vi "Configuration Keys.vi"(8 "error in":errorcluster, 11 "PowerSupply in":refnum<class "PowerSupply.lvclass">) -> (0 "error out":errorcluster, 2 "Required Keys":string[](array[string]), 3 "PowerSupply out":refnum<class "PowerSupply.lvclass">)   [LabVIEW 2019, in "PowerSupply.lvlib" / "PowerSupply.lvclass"]
doc: "Configuration Keys is a dynamic dispatch VI that reads a full inheritance chain's required key list.\n\nThis means each instrument must override this vi, and call the parent method . The end result is a comprehensive list of required keys that must be present in an instrument's config.ini file to correctly function."
uses:
  Library/PowerSupply.lvclass
  Custom Controls/Configuration Keys.ctl
  builds/Instruments/Instruments.lvlibp/Library/Instruments.lvclass
panel:
  in  "Configuration Keys":T1=enum."Number of Channels"
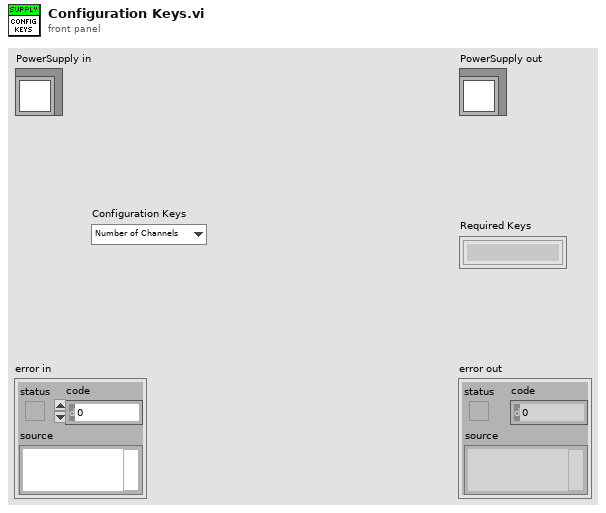
[diagram p1: front panel]
types:
  T1 = typedef "PowerSupply.lvlib/PowerSupply.lvclass/Configuration Keys.ctl" = enum16{"Is UUT Supply", "Number of Channels", "Channel Names", "Max Voltage", "Max Current", "Max OVP", "Max OCP", "Max Volt Ramp", "Max Curr Ramp"}
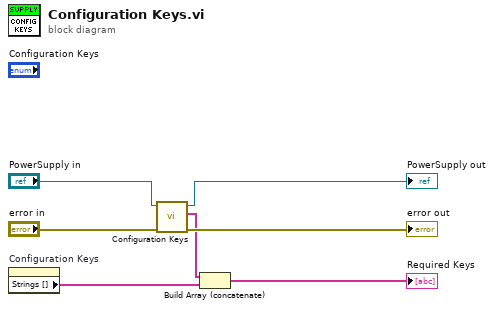
[diagram p0: block diagram]
diagram:
  n1 = property on="Configuration Keys" class="Enum (strict)"() -> ("Strings []"=w1:string[])  [unwired: 2 in, 2 out]
  n2 = call-parent "Configuration Keys.vi"("error in"="error in", "Instruments in"="PowerSupply in") -> ("error out"=→"error out":errorcluster, "Required Keys"=w3:string[], "Instruments out"=→"PowerSupply out":refnum<class "PowerSupply.lvclass">)  [unwired: 7 in]
  n3 = Build Array (concatenate)(w3, w1) -> (→"Required Keys":string[])
